vi "Characterizator.vi"(8 "error in (no error)":errorcluster, 11 "Main VI refnums":T4) -> (0 "Error out":errorcluster)   [LabVIEW 2016]
uses:
  Typedefs/Hit chart cluster refnum.ctl
  Typedefs/HitChart refnum.ctl
  <vilib>/Analysis/NI_AALBase.lvlib
panel:
  out "Waveform Chart":T1(graph)
  in  "Tab Control":enum32{"Page 1", "Page 2"}(tab)
  in  "Chnls":enum16{"Chnl 2", "Chnl 1", "Both"}(ring)=enum."Both"
  in  "Begin characterization":bool
  in  "Range max hard":dbl format="%#_g mV"
  in  "Range min hard":dbl format="%#_g mV"
  in  "Levels":i32
  in  "Save path":path=path "D:/Data/Characterizations/Coincidence rate characterizations"
  in  "Scintillator ID":i32
  in  "MPPC Serial number":i32
  in  "ROB 1 ID":i32 caption="ROB ID"
  in  "MPPC Bias":dbl
  in  "Recommended at 25C":bool
  in  "finish level":bool
  out "Current\n trigger level":dbl
  out "Level number":i32
  out "Datapoints ch1":i32
  out "Trigger level \nincrement":dbl
  out "Previous\n trigger level":dbl
  out "Ch1WaveformData":T2
  in  "Scintillator ID":i32
  in  "MPPC Serial number":i32
  in  "ROB 2 ID":i32 caption="ROB ID"
  in  "MPPC Bias":dbl
  in  "Recommended at 25C":bool
  in  "Channel 1":u8 max=15
  in  "Channel 2":u8=1 max=15
  in  "Register for channel events":bool
  out "Ch2WaveformData":T2
  in  "Hard-set trig lvl":bool=TRUE
  in  "Range max perc.":dbl min=0.0 max=100.0 format="%#_g %"
  in  "Range min perc.":dbl min=0.0 max=100.0 format="%#_g %"
  out "Datapoints ch2":i32
  in  "Datapoints to collect":i32=15
  in  "Period (s)":dbl=1.0 format="%#_13g"
  in  "Window(ns)":i32=5
  in  "stop":bool
  out "Command Queue":string[](array[string])
  in  "Data ch1":i32[][](array[numeric])
  out "Range max ref":refnum<vi>
  out "Range min ref":refnum<vi>
  in  "Data ch2":i32[][](array[numeric])
  out "Take data":bool
  in  "generate error":bool
  # "Channel 1"
  # "Channel 2"
  # "(Make sure they match main VI...)"
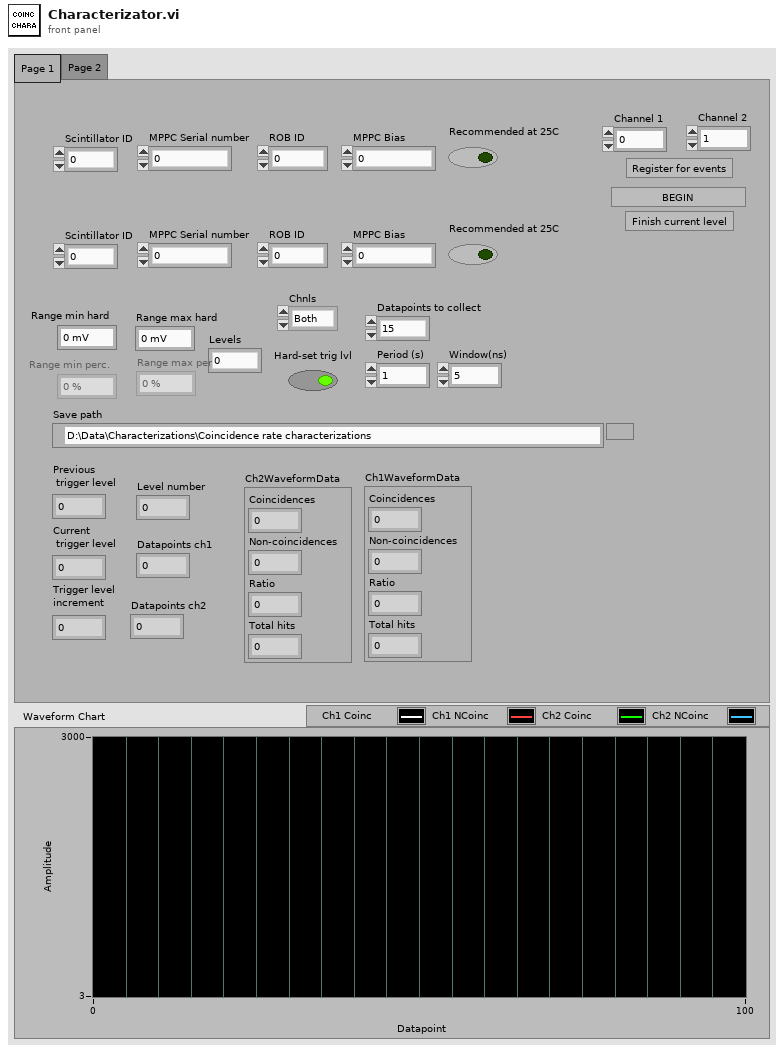
[diagram p1: front panel]
types:
  T1 = cluster{"Ch1 coinc":dbl, "Ch1 Ncoinc":dbl, "Ch2 coinc":dbl, "Ch2 Ncoinc":dbl}
  T2 = cluster{"Coincidences":dbl, "Non-coincidences":dbl, "Ratio":dbl, "Total hits":dbl}
  T3 = typedef "Hit chart cluster refnum.ctl" = refnum<vi>
  T4 = cluster{"VTrig mV":refnum<vi>, "Top hit charts":T3, "Bottom hit charts":T3, "Board selector":refnum<vi>, "VTrig percent ":refnum<vi>, "Hard-set value":refnum<vi>, "Programmatic set trigthres":refnum<vi>}
  T5 = enum16{"open", "replace", "create", "open or create", "replace or create", "replace or create with confirmation"}
  T6 = cluster{"Coincidences":dbl, "Non-coincidences":dbl, "Ratio":dbl, "Total hits":dbl}[]
  T7 = typedef "HitChart refnum.ctl" = refnum<vi>
  T8 = enum8{"Enabled", "Disabled", "Disabled and Grayed Out"}
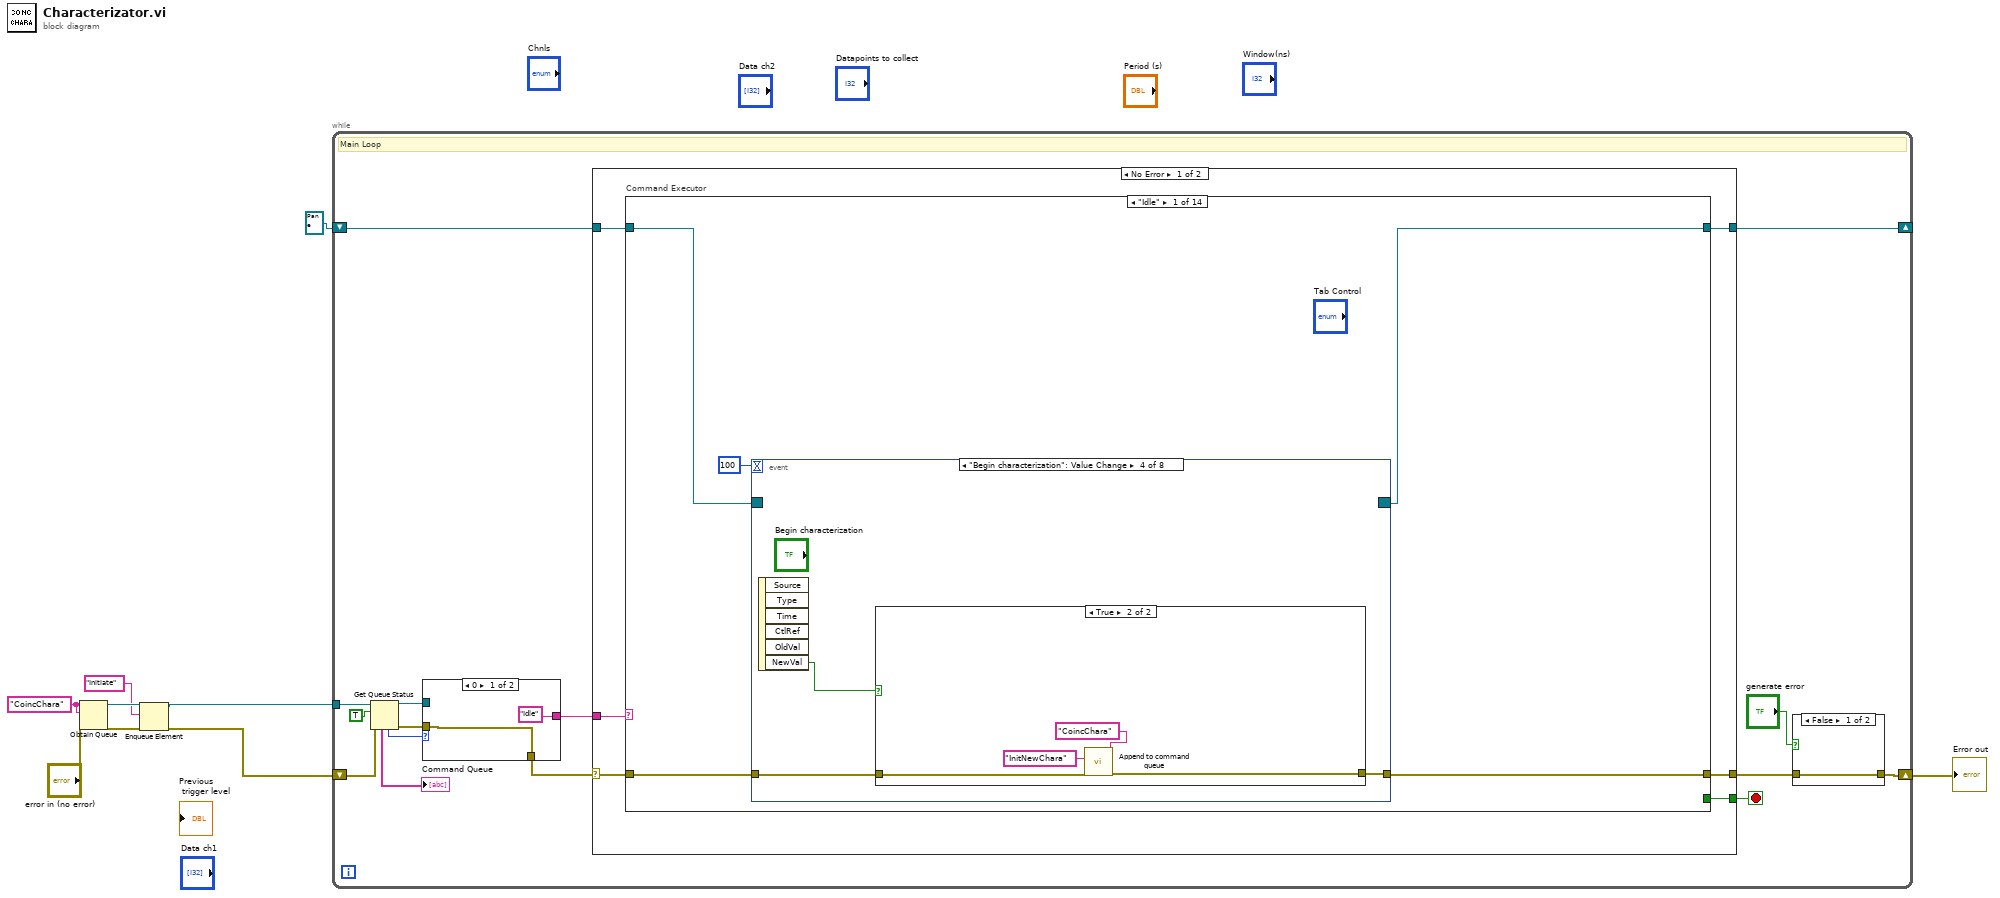
[diagram p0: block diagram]
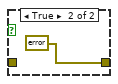
[diagram p2: hidden frame]
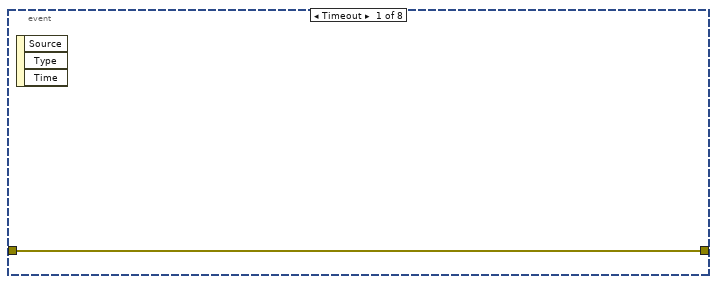
[diagram p3: hidden frame]
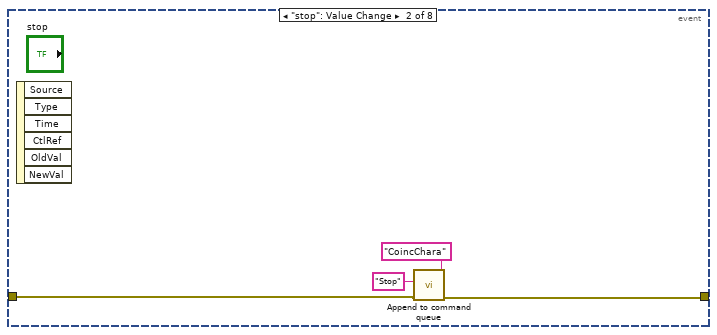
[diagram p4: hidden frame]
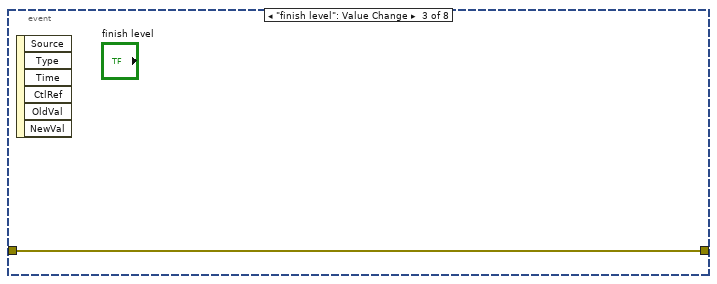
[diagram p5: hidden frame]
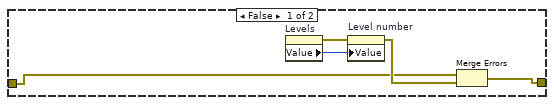
[diagram p6: hidden frame]
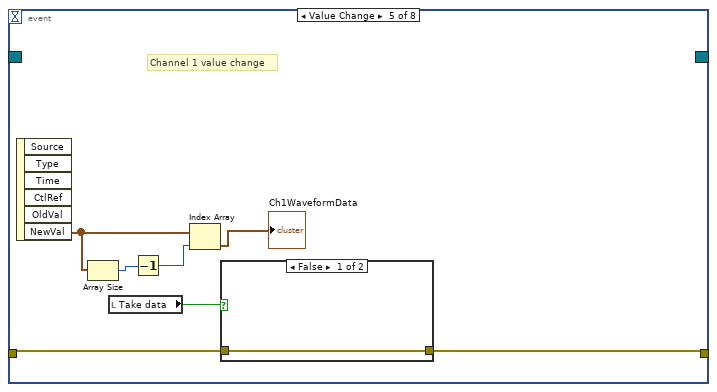
[diagram p7: hidden frame]
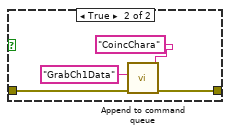
[diagram p8: hidden frame]
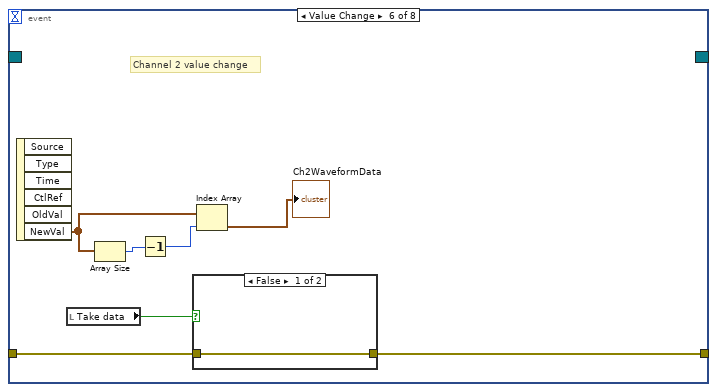
[diagram p9: hidden frame]
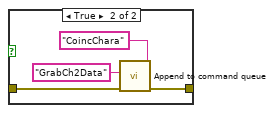
[diagram p10: hidden frame]
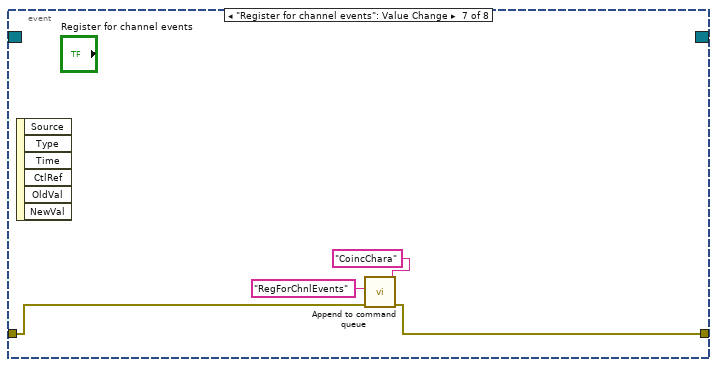
[diagram p11: hidden frame]
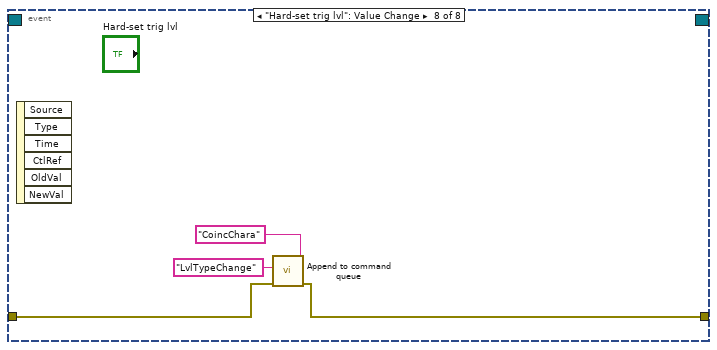
[diagram p12: hidden frame]
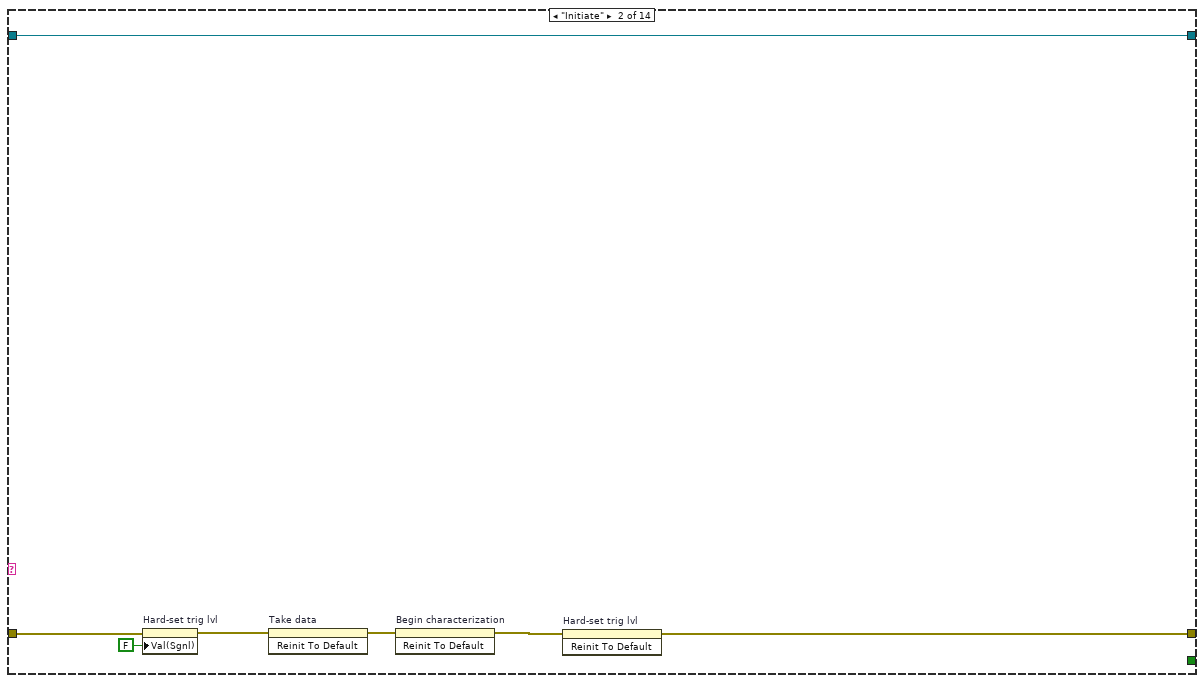
[diagram p13: hidden frame]
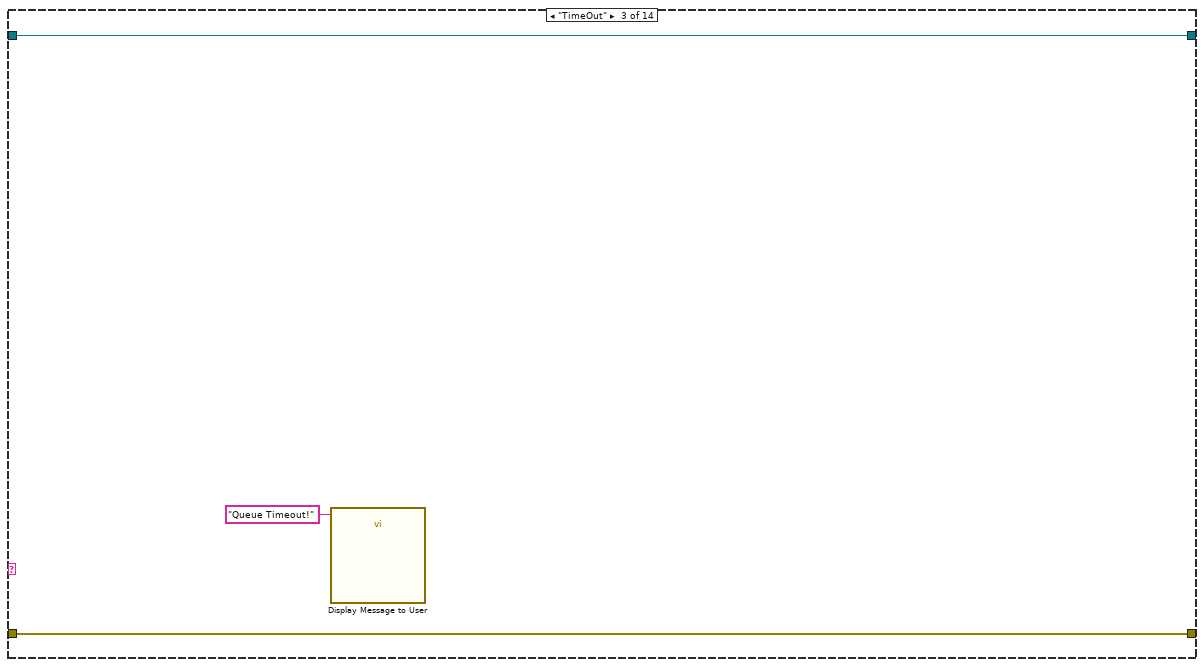
[diagram p14: hidden frame]
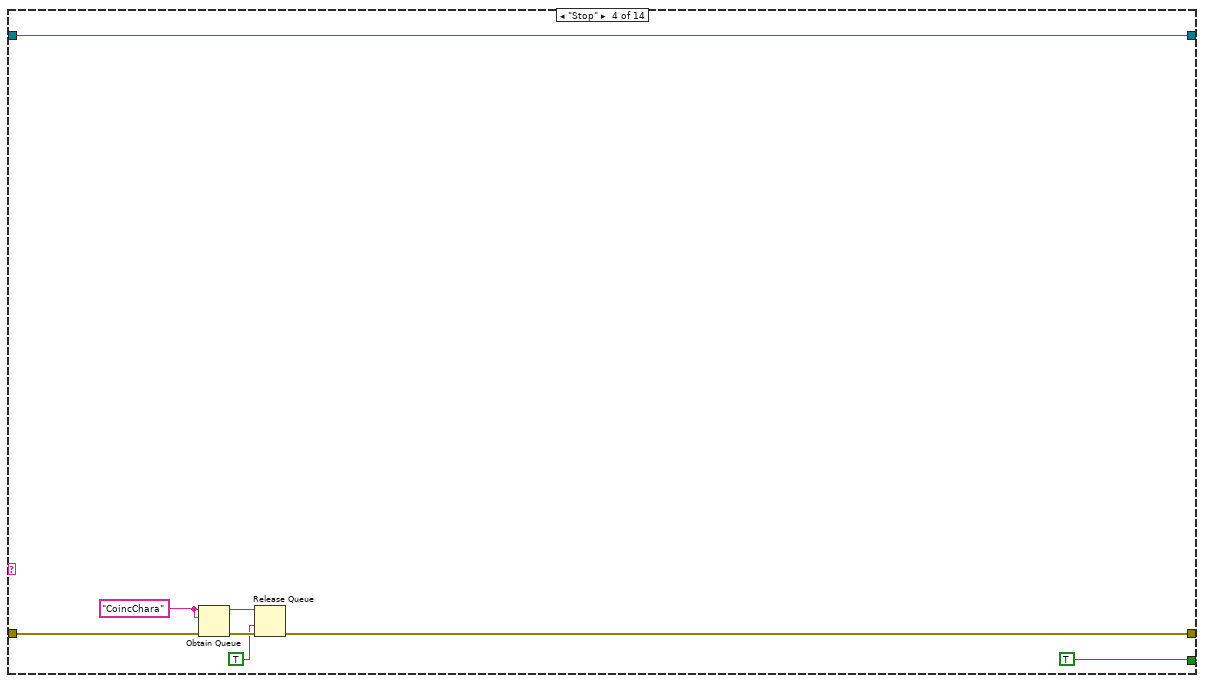
[diagram p15: hidden frame]
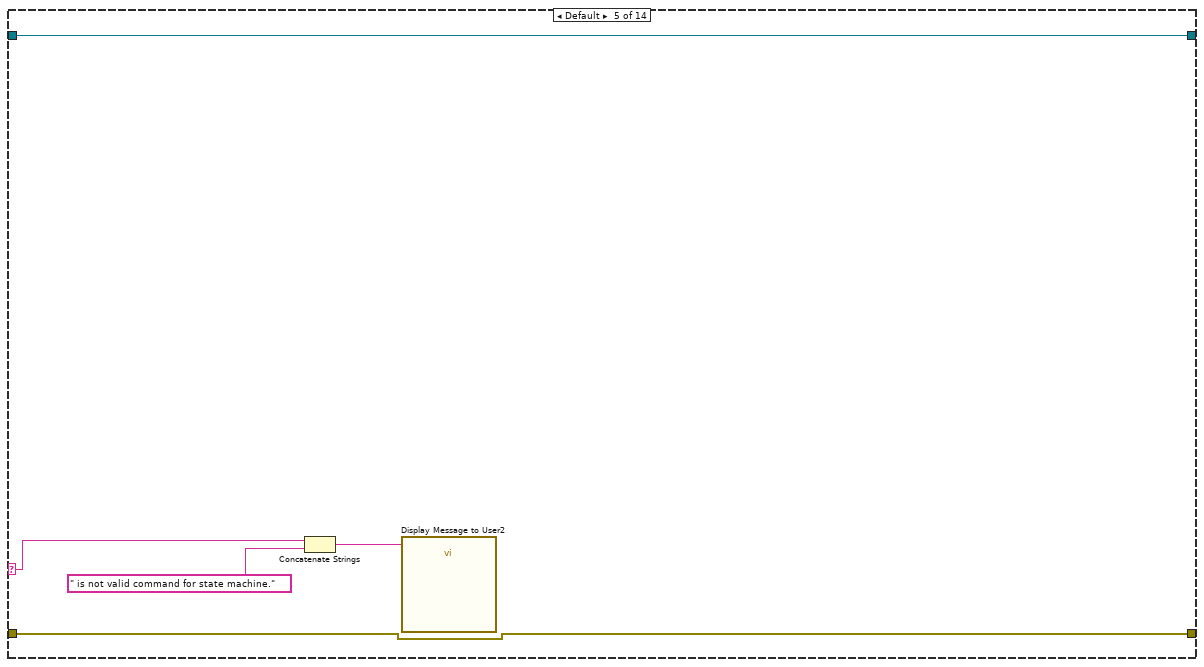
[diagram p16: hidden frame]
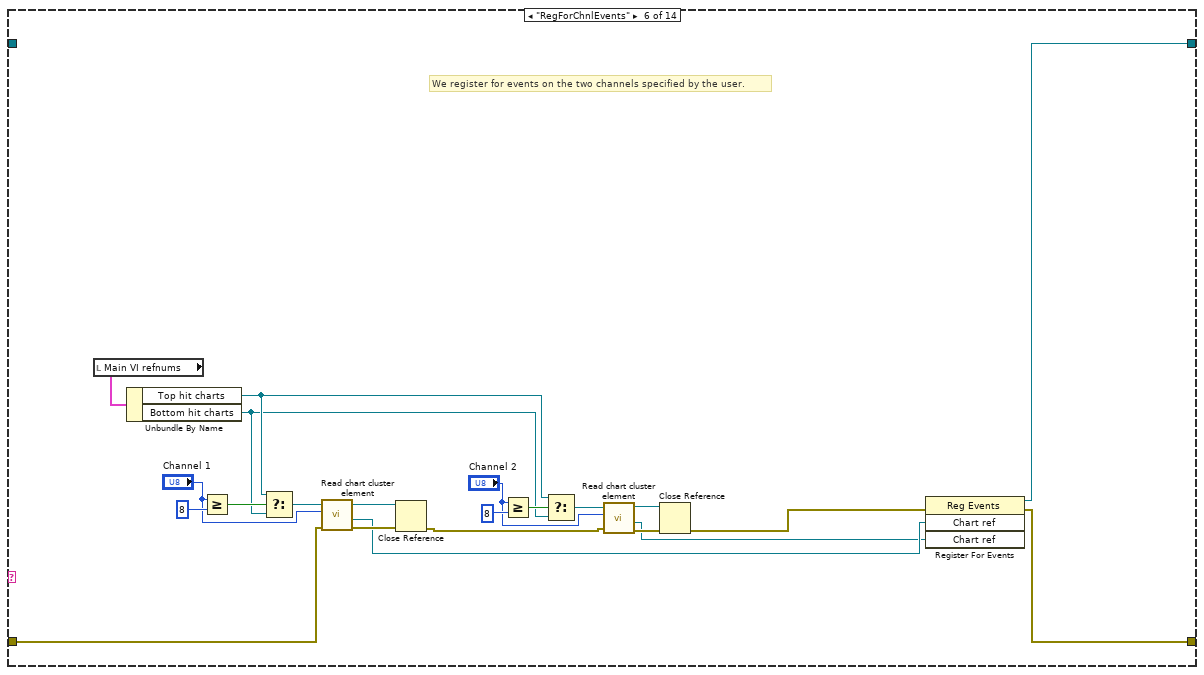
[diagram p17: hidden frame]
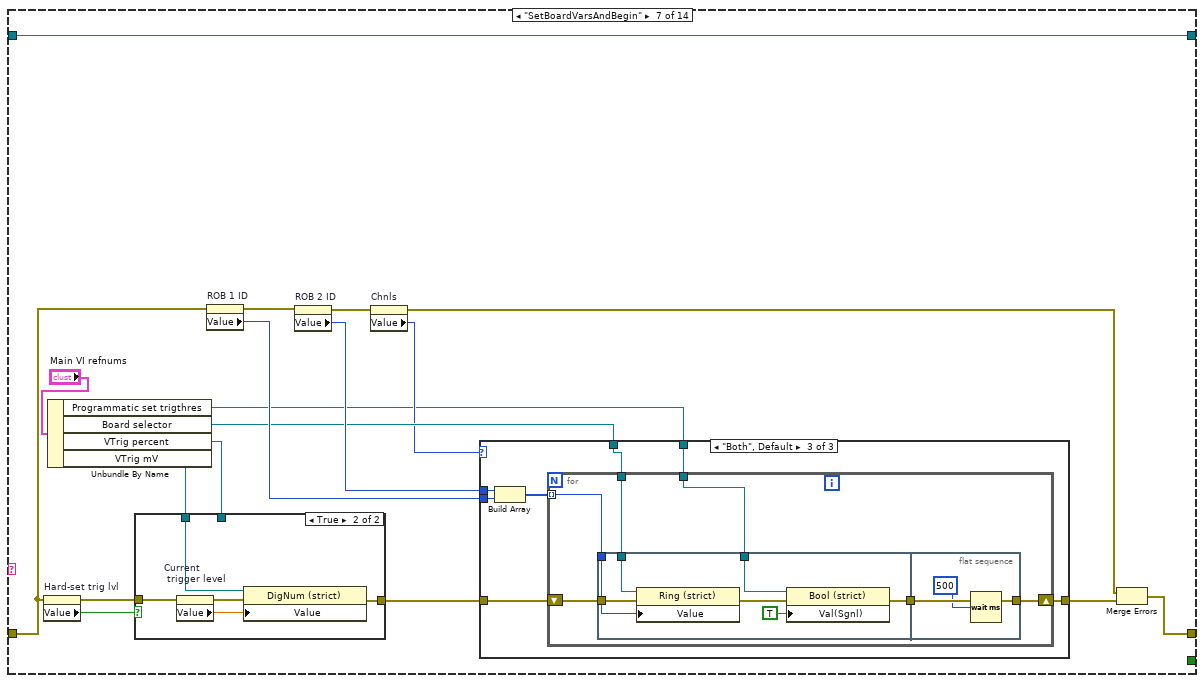
[diagram p18: hidden frame]
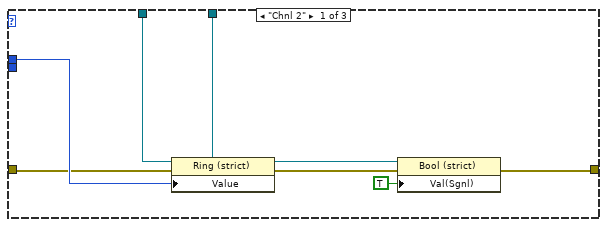
[diagram p19: hidden frame]
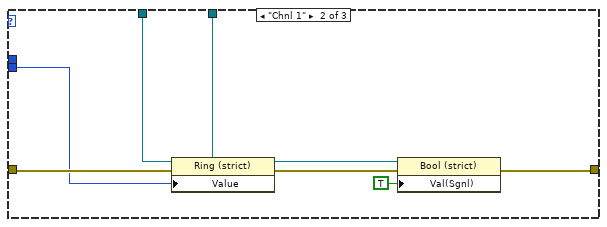
[diagram p20: hidden frame]
diagram:
  w9 = "CoincChara" ("name (unnamed)")
  n1 = Obtain Queue(name (unnamed)=w9, element data type=w9, error in (no error)="error in (no error)") -> (queue out=w7:refnum<queue>, error out=w5:errorcluster)  [unwired: 2 in, 1 out]
  n2 = Enqueue Element(queue=w7, element="Initiate", error in (no error)=w5) -> (queue out=w3:refnum<queue>, error out=w4:errorcluster)  [unwired: 1 in, 1 out]
  n3 = while {
    tunnel: w3 -> [w20]
    shift-right: [w12] -> w2
    shift-left: w4 -> [w17]
    shift-right: [w13] -> _
    shift-left: refnum<event-registration> refnum ("event registration refnum") -> [w14]
    stop <- w16 stop-if-true
    # "Main Loop"
    n4 = Get Queue Status(queue=w20, return elements? (F)=TRUE, error in (no error)=w17) -> (queue out=w23:refnum<queue>, error out=w22:errorcluster, # elements in queue=w24:i32, elements=→"Command Queue":string[])  [unwired: 4 out]
    n5 = case shown="0" w24 {
      tunnel: ["Idle" ("element") w510] -> w18
      tunnel: w23 -> [_ w516]
      tunnel: w22 -> [w506 w515]
      tunnel: [w506 w509] -> w15
      frame 0 {
      }
      frame Default {
        n6 = Dequeue Element(queue=w516, timeout in ms (-1)=50, error in (no error)=w515) -> (element=w514:string, timed out?=w513:bool, error out=w509:errorcluster)  [unwired: 1 out]
        n7 = Not(x=w513) -> (.not. x?=w512:bool)
        n8 = Select(t=w514, s=w512, f="TimeOut") -> (s? t:f=w510:string)
      }
    }
    n9 = case shown="No Error" w15 {
      selector: w15 -> [w29 w499]
      tunnel: w18 -> [w32 _]
      tunnel: [w31 w498] -> w11
      tunnel: [w30 TRUE] -> w16
      tunnel: w14 -> [w28 w495]
      tunnel: [w27 w495] -> w13
      frame No Error {
        n10 = case "Command Executor" shown="\"Idle\"" w32 {
          selector: w32 -> [_ _ _ _ w108 _ _ _ _ _ _ _ _ _]
          tunnel: [w35 w88 w96 w99 w107 w115 w141 w211 w225 w317 w374 w391 w406 w450] -> w31
          tunnel: w29 -> [w36 w92 w96 w100 w107 w116 w143 w200 w227 w271 w381 w394 w422 w467]
          tunnel: [_ _ _ TRUE _ _ _ _ _ _ _ _ _ _] -> w30
          tunnel: w28 -> [w34 w94 w95 w98 w106 _ w150 w208 w217 w314 w379 w404 w418 w463]
          tunnel: [w33 w94 w95 w98 w106 w114 w150 w208 w217 w314 w379 w404 w418 w463] -> w27
          frame "Idle" {
            n11 = event shown="[3] \"Begin characterization\": Value Change" {
              selector: w34 -> [_ _ _ _ _ _ _ _]
              dyn-events: [_ _ _ _ _ _ _ _] -> w33
              timeout: 100 -> [_ _ _ _ _ _ _ _]
              tunnel: w36 -> [w38 w42 w43 w46 w62 w74 w81 w86]
              tunnel: [w38 w41 w43 w45 w61 w73 w80 w85] -> w35
              event Timeout {
                n12 = event-data() -> ()  [unwired: 1 in, 3 out]
              }
              event "stop": Value Change {
                n13 = event-data() -> ()  [unwired: 1 in, 6 out]
                n14 = call "Append to command queue.vi"("Name (CommandQueue)"="CoincChara", "error in (no error)"=w42, "Single command"="Stop") -> ("error out"=w41:errorcluster)  [unwired: 8 in]
              }
              event "finish level": Value Change {
                n15 = event-data() -> ()  [unwired: 1 in, 6 out]
              }
              event "Begin characterization": Value Change {
                n16 = event-data() -> ("NewVal"=w44:bool)  [unwired: 1 in, 5 out]
                n17 = case shown="True" w44 {
                  tunnel: w46 -> [w47 w54]
                  tunnel: [w48 w53] -> w45
                  frame False {
                    n18 = property on="Levels" class="DigNum (strict)"() -> (error out=w50:errorcluster, "Value"=w51:i32)  [unwired: 2 in, 1 out]
                    n19 = property on="Level number" class="DigNum (strict)"(error in=w50, "Value"=w51) -> (error out=w49:errorcluster)  [unwired: 1 in, 1 out]
                    n20 = Merge Errors(w47, w49) -> (w48:errorcluster)
                  }
                  frame True {
                    n21 = call "Append to command queue.vi"("Name (CommandQueue)"="CoincChara", "error in (no error)"=w54, "Single command"="InitNewChara") -> ("error out"=w53:errorcluster)  [unwired: 8 in]
                  }
                }
              }
              event Value Change {
                # "Channel 1 value change"
                n22 = event-data() -> ("NewVal"=w58:T6)  [unwired: 1 in, 5 out]
                n23 = Array Size(array=w58) -> (size(s)=w57:i32)
                n24 = local read "Take data"() -> (w60:bool)
                n25 = Decrement(x=w57) -> (x-1=w56:i32)
                n26 = Index Array(array=w58, index=w56) -> (element=→"Ch1WaveformData":T2)
                n27 = case shown="False" w60 {
                  tunnel: w62 -> [w63 w65]
                  tunnel: [w63 w64] -> w61
                  frame False {
                  }
                  frame True {
                    n28 = call "Append to command queue.vi"("Name (CommandQueue)"="CoincChara", "error in (no error)"=w65, "Single command"="GrabCh1Data") -> ("error out"=w64:errorcluster)  [unwired: 8 in]
                  }
                }
              }
              event Value Change {
                # "Channel 2 value change"
                n29 = event-data() -> ("NewVal"=w69:T6)  [unwired: 1 in, 5 out]
                n30 = local read "Take data"() -> (w72:bool)
                n31 = Array Size(array=w69) -> (size(s)=w71:i32)
                n32 = Decrement(x=w71) -> (x-1=w70:i32)
                n33 = case shown="False" w72 {
                  tunnel: w74 -> [w75 w78]
                  tunnel: [w75 w77] -> w73
                  frame False {
                  }
                  frame True {
                    n34 = call "Append to command queue.vi"("Name (CommandQueue)"="CoincChara", "error in (no error)"=w78, "Single command"="GrabCh2Data") -> ("error out"=w77:errorcluster)  [unwired: 8 in]
                  }
                }
                n35 = Index Array(array=w69, index=w70) -> (element=→"Ch2WaveformData":T2)
              }
              event "Register for channel events": Value Change {
                n36 = event-data() -> ()  [unwired: 1 in, 6 out]
                n37 = call "Append to command queue.vi"("Name (CommandQueue)"="CoincChara", "error in (no error)"=w81, "Single command"="RegForChnlEvents") -> ("error out"=w80:errorcluster)  [unwired: 8 in]
              }
              event "Hard-set trig lvl": Value Change {
                n38 = event-data() -> ()  [unwired: 1 in, 6 out]
                n39 = call "Append to command queue.vi"("Name (CommandQueue)"="CoincChara", "error in (no error)"=w86, "Single command"="LvlTypeChange") -> ("error out"=w85:errorcluster)  [unwired: 8 in]
              }
            }
          }
          frame "Initiate" {
            n40 = property on="Hard-set trig lvl" class="Bool (strict)"(error in=w92, "Val(Sgnl)"=FALSE ("Value (Signaling)")) -> (error out=w91:errorcluster)  [unwired: 1 in, 1 out]
            n41 = invoke on="Take data" class="Bool (strict)" method="Reinit To Default"(error in=w91) -> (error out=w90:errorcluster)  [unwired: 2 in, 2 out]
            n42 = invoke on="Begin characterization" class="Bool (strict)" method="Reinit To Default"(error in=w90) -> (error out=w89:errorcluster)  [unwired: 2 in, 2 out]
            n43 = invoke on="Hard-set trig lvl" class="Bool (strict)" method="Reinit To Default"(error in=w89) -> (error out=w88:errorcluster)  [unwired: 2 in, 2 out]
          }
          frame "TimeOut" {
            n44 = call "Display Message to User"("Message"="Queue Timeout!" ("string")) -> ()  [unwired: 9 in, 2 out]
          }
          frame "Stop" {
            w101 = "CoincChara" ("name (unnamed)")
            n45 = Obtain Queue(name (unnamed)=w101, element data type=w101, error in (no error)=w100) -> (queue out=w104:refnum<queue>, error out=w103:errorcluster)  [unwired: 2 in, 1 out]
            n46 = Release Queue(queue=w104, force destroy? (F)=TRUE, error in (no error)=w103) -> (error out=w99:errorcluster)  [unwired: 2 out]
          }
          frame Default {
            n47 = Concatenate Strings(w108, " is not valid command for state machine." ("string")) -> (w109:string)
            n48 = call "Display Message to User2"("Message"=w109) -> ()  [unwired: 9 in, 2 out]
          }
          frame "RegForChnlEvents" {
            # "We register for events on the two channels specified by the user."
            n49 = local read "Main VI refnums"() -> (w113:T4)
            n50 = Unbundle By Name(w113) -> ("Top hit charts"=w112:T3, "Bottom hit charts"=w111:T3)
            n51 = Greater Or Equal?(x="Channel 1", y=u8 8) -> (x >= y?=w131:bool)
            n52 = Select(t=w112, s=w131, f=w111) -> (s? t:f=w130:T3)
            n53 = call "Read chart cluster element.vi"("error in (no error)"=w116, "Channel"="Channel 1", "Chart cluster"=w130) -> ("error out"=w124:errorcluster, "Chart ref"=w118:T7, "Chart cluster"=w123:T3)  [unwired: 5 in, 1 out]
            n54 = Close Reference(reference=w123, error in (no error)=w124) -> (error out=w122:errorcluster)
            n55 = Greater Or Equal?(x="Channel 2", y=u8 8) -> (x >= y?=w127:bool)
            n56 = Select(t=w112, s=w127, f=w111) -> (s? t:f=w128:T3)
            n57 = call "Read chart cluster element.vi"("error in (no error)"=w122, "Channel"="Channel 2", "Chart cluster"=w128) -> ("error out"=w121:errorcluster, "Chart ref"=w117:T7, "Chart cluster"=w119:T3)  [unwired: 5 in, 1 out]
            n58 = Close Reference(reference=w119, error in (no error)=w121) -> (error out=w120:errorcluster)
            n59 = register-events(error in=w120, w118, w117) -> (reference out=w114:refnum<event-registration>, error out=w115:errorcluster)  [unwired: 1 in]
          }
          frame "SetBoardVarsAndBegin" {
            n60 = property on="Hard-set trig lvl" class="Bool (strict)"(error in=w143) -> (error out=w147:errorcluster, "Value"=w148:bool)  [unwired: 1 in, 1 out]
            n61 = Unbundle By Name("Main VI refnums") -> ("Programmatic set trigthres"=w133:refnum<vi>, "Board selector"=w140:refnum<vi>, "VTrig percent"=w139:refnum<vi>, "VTrig mV"=w138:refnum<vi>)
            n62 = case shown="True" w148 {
              tunnel: [w189 w194] -> w149
              tunnel: w147 -> [w188 w193]
              tunnel: w139 -> [w187 _]
              tunnel: w138 -> [_ w192]
              frame False {
                n63 = property on="Current\n trigger level" class="DigNum (strict)"(error in=w188) -> (error out=w190:errorcluster, "Value"=w191:dbl)  [unwired: 1 in, 1 out]
                n64 = property class="DigNum (strict)"(reference=w187, error in=w190, "Value"=w191) -> (error out=w189:errorcluster)  [unwired: 1 out]
              }
              frame True {
                n65 = property on="Current\n trigger level" class="DigNum (strict)"(error in=w193) -> (error out=w195:errorcluster, "Value"=w196:dbl)  [unwired: 1 in, 1 out]
                n66 = property class="DigNum (strict)"(reference=w192, error in=w195, "Value"=w196) -> (error out=w194:errorcluster)  [unwired: 1 out]
              }
            }
            n67 = property on="ROB 1 ID" class="DigNum (strict)"(error in=w143) -> (error out=w146:errorcluster, "Value"=w144:i32)  [unwired: 1 in, 1 out]
            n68 = property on="ROB 2 ID" class="DigNum (strict)"(error in=w146) -> (error out=w137:errorcluster, "Value"=w145:i32)  [unwired: 1 in, 1 out]
            n69 = property on="Chnls" class="Enum (strict)"(error in=w137) -> (error out=w136:errorcluster, "Value"=w135:enum16{"Chnl 2", "Chnl 1", "Both"})  [unwired: 1 in, 1 out]
            n70 = case shown="\"Both\", Default" w135 {
              tunnel: w149 -> [w151 w159 w171]
              tunnel: w145 -> [w152 _ w170]
              tunnel: w144 -> [_ w158 w169]
              tunnel: [w155 w162 w167] -> w142
              tunnel: w140 -> [w153 w160 w166]
              tunnel: w133 -> [w154 w161 w165]
              frame "Chnl 2" {
                n71 = property class="Ring (strict)"(reference=w153, error in=w151, "Value"=w152) -> (error out=w156:errorcluster)  [unwired: 1 out]
                n72 = property class="Bool (strict)"(reference=w154, error in=w156, "Val(Sgnl)"=TRUE ("Value (Signaling)")) -> (error out=w155:errorcluster)  [unwired: 1 out]
              }
              frame "Chnl 1" {
                n73 = property class="Ring (strict)"(reference=w160, error in=w159, "Value"=w158) -> (error out=w163:errorcluster)  [unwired: 1 out]
                n74 = property class="Bool (strict)"(reference=w161, error in=w163, "Val(Sgnl)"=TRUE ("Value (Signaling)")) -> (error out=w162:errorcluster)  [unwired: 1 out]
              }
              frame "Both", Default {
                n75 = Build Array(w170, w169) -> (w168:i32[])
                n76 = for {
                  tunnel: w166 -> [w175]
                  tunnel: w165 -> [w174]
                  tunnel: w168 -> [w173] mode=indexing
                  shift-right: [w177] -> w167
                  shift-left: w171 -> [w176]
                  n77 = flat-sequence {
                    tunnel: w176 -> [w182]
                    tunnel: w175 -> [w180]
                    tunnel: w174 -> [w179]
                    tunnel: w173 -> [w178]
                    tunnel: [w183] -> w172
                    tunnel: [w186] -> w177
                    tunnel: w172 -> [w186]
                    frame #0 {
                      n78 = property class="Ring (strict)"(reference=w180, error in=w182, "Value"=w178) -> (error out=w181:errorcluster)  [unwired: 1 out]
                      n79 = property class="Bool (strict)"(reference=w179, error in=w181, "Val(Sgnl)"=TRUE ("Value (Signaling)")) -> (error out=w183:errorcluster)  [unwired: 1 out]
                    }
                    frame #1 {
                      n80 = Wait (ms)(milliseconds to wait=500) -> ()  [unwired: 1 out]
                    }
                  }
                }
              }
            }
            n81 = Merge Errors(w136, w142) -> (w141:errorcluster)
          }
          frame "InitNewChara" {
            w198 = -2 ("Datapoints")
            n82 = property on="Range min ref" class="LVObjRef (strict)"(error in=w200) -> (error out=w203:errorcluster, "Value"=w204:refnum<vi>)  [unwired: 1 in, 1 out]
            n83 = property class="DigNum (strict)"(reference=w204, error in=w203) -> (error out=w201:errorcluster, "Value"=w206:dbl)  [unwired: 1 out]
            n84 = property on="Range max ref" class="LVObjRef (strict)"(error in=w201) -> (error out=w202:errorcluster, "Value"=w205:refnum<vi>)  [unwired: 1 in, 1 out]
            n85 = property class="DigNum (strict)"(reference=w205, error in=w202) -> (error out=w199:errorcluster, "Value"=w207:dbl)  [unwired: 1 out]
            "Current\n trigger level" <- w207
            n86 = Decrement(x="Levels") -> (x-1=w209:i32)
            n87 = local write "Take data"(TRUE ("Take data")) -> ()
            n88 = Subtract(x=w207, y=w206) -> (x-y=w215:dbl)
            n89 = Divide(x=w215, y=w209) -> (x/y=→"Trigger level \nincrement":dbl)
            n90 = call "Append to command queue.vi"("Name (CommandQueue)"="CoincChara", "error in (no error)"=w199, "Single command"="SetBoardVarsAndBegin") -> ("error out"=w211:errorcluster)  [unwired: 8 in]
            "Level number" <- 1 ("Level number")
            "Datapoints ch1" <- w198
            "Datapoints ch2" <- w198
          }
          frame "LevelDone" {
            n91 = property on="Levels" class="DigNum (strict)"(error in=w227) -> (error out=w228:errorcluster, "Value"=w229:i32)  [unwired: 1 in, 1 out]
            n92 = property on="Level number" class="DigNum (strict)"(error in=w228) -> (error out=w222:errorcluster, "Value"=w230:i32)  [unwired: 1 in, 1 out]
            n93 = Equal?(x=w230, y=w229) -> (x = y?=w226:bool)
            n94 = call "Append to command queue.vi"("Name (CommandQueue)"="CoincChara", "error in (no error)"=w222, "Single command"="SaveData") -> ("error out"=w219:errorcluster)  [unwired: 8 in]
            n95 = property on="Current\n trigger level" class="DigNum (strict)"(error in=w219) -> (error out=w220:errorcluster, "Value"=w221:dbl)  [unwired: 1 in, 1 out]
            n96 = property on="Previous\n trigger level" class="DigNum (strict)"(error in=w220, "Value"=w221) -> (error out=w218:errorcluster)  [unwired: 1 in, 1 out]
            n97 = case shown="False" w226 {
              tunnel: w218 -> [w241 w251]
              tunnel: [w231 w250] -> w225
              frame False {
                w236 = -2 ("Datapoints ch1")
                n98 = property on="Trigger level \nincrement" class="DigNum (strict)"(error in=w241) -> (error out=w245:errorcluster, "Value"=w244:dbl)  [unwired: 1 in, 1 out]
                n99 = property on="Current\n trigger level" class="DigNum (strict)"(error in=w245) -> (error out=w242:errorcluster, "Value"=w237:dbl)  [unwired: 1 in, 1 out]
                n100 = Subtract(x=w237, y=w244) -> (x-y=w243:dbl)
                n101 = property on="Current\n trigger level" class="DigNum (strict)"(error in=w242, "Value"=w243) -> (error out=w234:errorcluster)  [unwired: 1 in, 1 out]
                n102 = property on="Level number" class="DigNum (strict)"(error in=w234) -> (error out=w246:errorcluster, "Value"=w248:i32)  [unwired: 1 in, 1 out]
                n103 = property on="Datapoints ch1" class="DigNum (strict)"(error in=w234, "Value"=w236) -> (error out=w235:errorcluster)  [unwired: 1 in, 1 out]
                n104 = property on="Datapoints ch2" class="DigNum (strict)"(error in=w235, "Value"=w236) -> (error out=w233:errorcluster)  [unwired: 1 in, 1 out]
                n105 = Increment(x=w248) -> (x+1=w247:i32)
                n106 = property on="Level number" class="DigNum (strict)"(error in=w246, "Value"=w247) -> (error out=w238:errorcluster)  [unwired: 1 in, 1 out]
                n107 = call "Append to command queue.vi"("Name (CommandQueue)"="CoincChara", "error in (no error)"=w238, "Single command"="SetBoardVarsAndBegin") -> ("error out"=w232:errorcluster)  [unwired: 8 in]
                n108 = Merge Errors(w232, w233) -> (w231:errorcluster)
              }
              frame True {
                n109 = call "Append to command queue.vi"("Name (CommandQueue)"="CoincChara", "error in (no error)"=w251, "Single command"="Reset") -> ("error out"=w250:errorcluster)  [unwired: 8 in]
              }
            }
          }
          frame "SaveData" {
            w275 = i32[][] [] ("Data")
            n110 = property on="Period (s)" class="DigNum (strict)"(error in=w271) -> (error out=w294:errorcluster, "Value"=w295:dbl)  [unwired: 1 in, 1 out]
            n111 = property on="Previous\n trigger level" class="DigNum (strict)"(error in=w294) -> (error out=w277:errorcluster, "Value"=w296:dbl)  [unwired: 1 in, 1 out]
            n112 = property on="Hard-set trig lvl" class="Bool (strict)"(error in=w277) -> (error out=w254:errorcluster, "Value"=w285:bool)  [unwired: 1 in, 1 out]
            n113 = Number To Decimal String(number=w296) -> (decimal integer string=w311:string)  [unwired: 1 in]
            n114 = Number To Decimal String(number=w295) -> (decimal integer string=w315:string)  [unwired: 1 in]
            n115 = call "Build header single level.vi"("Overvoltage"="MPPC Bias", "Recommended at 25C"="Recommended at 25C", "MPPC Serial number"="MPPC Serial number", "ROB ID"="ROB 1 ID", "Scintillator ID"="Scintillator ID") -> ("Header"=w280:string)  [unwired: 6 in]
            n116 = Select(t="percent " ("string"), s=w285, f="mV " ("string")) -> (s? t:f=w286:string)
            n117 = Concatenate Strings(w311, w286, w315, "s.csv " ("string")) -> (w331:string)
            n118 = call "Build header single level.vi"("Overvoltage"="MPPC Bias", "Recommended at 25C"="Recommended at 25C", "Add timestamp"=FALSE, "MPPC Serial number"="MPPC Serial number", "ROB ID"="ROB 2 ID", "Scintillator ID"="Scintillator ID") -> ("Header"=w279:string)  [unwired: 5 in]
            n119 = Build Array(w280, w279) -> (w278:string[])
            n120 = Build Array("Ch1" ("string"), "Ch2" ("string")) -> (w281:string[])
            n121 = Select(t="Hardset" ("string"), s=w285, f="Percent" ("string")) -> (s? t:f=w291:string)
            n122 = Concatenate Strings("Trig lvl:  " ("string"), w291) -> (w289:string)
            n123 = property on="Data ch2" class="Arr (strict)"() -> (error out=w310:errorcluster, "Value"=w269:i32[][])  [unwired: 2 in, 1 out]
            n124 = property on="Data ch1" class="Arr (strict)"(error in=w310) -> (error out=w309:errorcluster, "Value"=w270:i32[][])  [unwired: 1 in, 1 out]
            n125 = Index Array(array=w270, index (col) #1=0 ("index (row)"), index (col) #2=1 ("index (row)")) -> (element #1=w268:i32[], element #2=w267:i32[])  [unwired: 2 in]
            n126 = Index Array(array=w269, index (col) #1=0 ("index (row)"), index (col) #2=1 ("index (row)")) -> (element #1=w266:i32[], element #2=w265:i32[])  [unwired: 2 in]
            n127 = Build Array(w270, w269) -> (w276:i32[][][])
            n128 = for {
              N: 2 -> [_]
              tunnel: "Save path" -> [w342]
              tunnel: w331 -> [w351]
              tunnel: w281 -> [w341] mode=indexing
              tunnel: w278 -> [w340] mode=indexing
              tunnel: w276 -> [w339] mode=indexing
              shift-right: [w343] -> w253
              shift-left: w254 -> [w337]
              n129 = Build Path(base path=w342, name or relative path=w341) -> (appended path=w338:path)
              n130 = call "Find or make folder.vi"("error in"=w337, "Folder to find/make"=w338) -> ("error out"=w336:errorcluster, "created path"=w335:path)  [unwired: 7 in, 1 out]
              n131 = Build Path(base path=w335, name or relative path=w351) -> (appended path=w353:path)
              n132 = Open/Create/Replace File(file path (use dialog)=w353, error in=w336, operation (0:open)=T5."open or create") -> (refnum out=w348:refnum<file>, error out=w347:errorcluster)  [unwired: 3 in, 1 out]
              n133 = Array To Spreadsheet String(delimiter (Tab)="\t", array=w339, 3:"%d" ("format string")) -> (spreadsheet string=w349:string)
              n134 = Concatenate Strings(w340, w349) -> (w346:string)
              n135 = Write to Text File(file (use dialog)=w348, text=w346, error in=w347) -> (refnum out=w345:refnum<file>, error out=w344:errorcluster)  [unwired: 1 in, 1 out]
              n136 = Close File(refnum=w345, error in=w344) -> (error out=w343:errorcluster)  [unwired: 1 out]
            }
            n137 = property on="Save path" class="Path"(error in=w253) -> (error out=w318:errorcluster, "Value"=w329:path)  [unwired: 1 in, 1 out]
            n138 = Build Path(base path=w329, name or relative path="Summary.csv") -> (appended path=w324:path)
            n139 = Open/Create/Replace File(file path (use dialog)=w324, error in=w318, operation (0:open)=T5."open") -> (refnum out=w327:refnum<file>, error out=w326:errorcluster)  [unwired: 3 in, 1 out]
            n140 = Unbundle By Name(w326) -> ("code"=w325:i32)
            n141 = case shown="7" w325 {
              tunnel: w327 -> [_ w372]
              tunnel: w326 -> [_ w371]
              tunnel: w324 -> [w364 _]
              tunnel: [w361 w367] -> w322
              tunnel: [w360 w366] -> w323
              tunnel: w279 -> [w357 _]
              tunnel: w280 -> [w356 _]
              tunnel: w289 -> [w355 _]
              frame 7 {
                w354 = "\r\n"
                n142 = call "Summary header gen.vi"() -> ("Header"=w358:string)
                n143 = Open/Create/Replace File(file path (use dialog)=w364, operation (0:open)=T5."create") -> (refnum out=w362:refnum<file>, error out=w363:errorcluster)  [unwired: 4 in, 1 out]
                n144 = Concatenate Strings(w356, w357, w358, w354, w355, w354) -> (w359:string)
                n145 = Write to Text File(file (use dialog)=w362, text=w359, error in=w363) -> (refnum out=w361:refnum<file>, error out=w360:errorcluster)  [unwired: 1 in, 1 out]
              }
              frame Default {
                n146 = Get File Size(file=w372, error in=w371) -> (refnum out=w370:refnum<file>, size (in bytes)=w369:i64, 0:w368:errorcluster)
                n147 = Set File Position(offset (in bytes) (0)=w369, refnum=w370, error in=w368) -> (refnum out=w367:refnum<file>, error out=w366:errorcluster)  [unwired: 1 in]
              }
            }
            n148 = call <vilib>:"Std Deviation and Variance.vi"("X"=w268) -> ("mean"=w263:dbl)  [unwired: 1 in, 2 out]
            n149 = call <vilib>:"Std Deviation and Variance.vi"("X"=w267) -> ("mean"=w262:dbl)  [unwired: 1 in, 2 out]
            n150 = call <vilib>:"Std Deviation and Variance.vi"("X"=w266) -> ("mean"=w261:dbl)  [unwired: 1 in, 2 out]
            n151 = call <vilib>:"Std Deviation and Variance.vi"("X"=w265) -> ("mean"=w260:dbl)  [unwired: 1 in, 2 out]
            n152 = property on="Period (s)" class="DigNum (strict)"(error in=w309) -> (error out=w308:errorcluster, "Value"=w313:dbl)  [unwired: 1 in, 1 out]
            n153 = Bundle By Name(cluster=T1 {"Ch1 coinc"=0.0, "Ch1 Ncoinc"=0.0, "Ch2 coinc"=0.0, "Ch2 Ncoinc"=0.0} ("Waveform Chart"), "Ch1 coinc"=w263, "Ch1 Ncoinc"=w262, "Ch2 coinc"=w261, "Ch2 Ncoinc"=w260) -> (→"Waveform Chart":T1)
            n154 = property on="Window(ns)" class="DigNum (strict)"(error in=w308) -> (error out=w272:errorcluster, "Value"=w312:i32)  [unwired: 1 in, 1 out]
            n155 = call "Data to sumamry.vi"("Window (ns)"=w312, "Period (seconds)"=w313, "Trig lvl"=w311, "ch2 data"=w269, "ch1 data"=w270) -> ("String out"=w321:string)  [unwired: 6 in]
            n156 = Write to Text File(file (use dialog)=w322, text=w321, error in=w323) -> (refnum out=w319:refnum<file>, error out=w320:errorcluster)  [unwired: 1 in, 1 out]
            n157 = property on="Data ch1" class="Arr (strict)"(error in=w272, "Value"=w275) -> (error out=w274:errorcluster)  [unwired: 1 in, 1 out]
            n158 = property on="Data ch2" class="Arr (strict)"(error in=w274, "Value"=w275) -> (error out=w273:errorcluster)  [unwired: 1 in, 1 out]
            n159 = Close File(refnum=w319, error in=w320) -> (error out=w316:errorcluster)  [unwired: 1 out]
            n160 = Merge Errors(w316, w273) -> (w317:errorcluster)
          }
          frame "Reset" {
            w377 = -2 ("Datapoints")
            n161 = property on="Level number" class="DigNum (strict)"(error in=w381, "Value"=1 ("Level number")) -> (error out=w380:errorcluster)  [unwired: 1 in, 1 out]
            n162 = property on="Datapoints ch1" class="DigNum (strict)"(error in=w380, "Value"=w377) -> (error out=w378:errorcluster)  [unwired: 1 in, 1 out]
            n163 = property on="Datapoints ch2" class="DigNum (strict)"(error in=w378, "Value"=w377) -> (error out=w375:errorcluster)  [unwired: 1 in, 1 out]
            n164 = property on="Begin characterization" class="Bool (strict)"(error in=w375, "Value"=FALSE ("Begin characterization")) -> (error out=w374:errorcluster)  [unwired: 1 in, 1 out]
            "Take data" <- FALSE ("Boolean")
          }
          frame "LvlTypeChange" {
            w399 = T8."Disabled and Grayed Out" ("Disabled")
            w400 = T8."Enabled" ("Disabled")
            n165 = property on="Hard-set trig lvl" class="Bool (strict)"(error in=w394) -> (error out=w398:errorcluster, "Value"=w395:bool)  [unwired: 1 in, 1 out]
            n166 = local read "Main VI refnums"() -> (w388:T4)
            n167 = Unbundle By Name(w388) -> ("Hard-set value"=w387:refnum<vi>)
            n168 = Select(t=w400, s=w395, f=w399) -> (s? t:f=w397:T8)
            n169 = property class="Bool (strict)"(reference=w387, error in=w394, "Val(Sgnl)"=w395) -> (error out=w392:errorcluster)  [unwired: 1 out]
            n170 = Select(t=w399, s=w395, f=w400) -> (s? t:f=w396:T8)
            n171 = control-ref of="Range max hard"() -> (w386:refnum<vi>)
            n172 = property class="DigNum (strict)"(reference=w386, error in=w398, "DisabledEnum"=w397) -> (error out=w403:errorcluster)  [unwired: 1 out]
            n173 = control-ref of="Range min hard"() -> (w383:refnum<vi>)
            n174 = property class="DigNum (strict)"(reference=w383, error in=w403, "DisabledEnum"=w397) -> (error out=w402:errorcluster)  [unwired: 1 out]
            n175 = control-ref of="Range max perc."() -> (w385:refnum<vi>)
            n176 = Select(t=w386, s=w395, f=w385) -> (s? t:f=→"Range max ref":refnum<vi>)
            n177 = property class="DigNum (strict)"(reference=w385, error in=w402, "DisabledEnum"=w396) -> (error out=w401:errorcluster)  [unwired: 1 out]
            n178 = control-ref of="Range min perc."() -> (w384:refnum<vi>)
            n179 = Select(t=w383, s=w395, f=w384) -> (s? t:f=→"Range min ref":refnum<vi>)
            n180 = property class="DigNum (strict)"(reference=w384, error in=w401, "DisabledEnum"=w396) -> (error out=w393:errorcluster)  [unwired: 1 out]
            n181 = Merge Errors(w392, w393) -> (w391:errorcluster)
          }
          frame "GrabCh1Data" {
            n182 = property on="Ch1WaveformData" class="Clust (strict)"(error in=w422) -> (error out=w421:errorcluster, "Value"=w420:T2)  [unwired: 1 in, 1 out]
            n183 = property on="Datapoints ch1" class="DigNum (strict)"(error in=w421) -> (error out=w414:errorcluster, "Value"=w411:i32)  [unwired: 1 in, 1 out]
            n184 = property on="Datapoints to collect" class="DigNum (strict)"(error in=w414) -> (error out=w410:errorcluster, "Value"=w412:i32)  [unwired: 1 in, 1 out]
            n185 = Equal?(x=w412, y=w411) -> (x = y?=w413:bool)
            n186 = case shown="True" w413 {
              tunnel: w411 -> [w433 w449]
              tunnel: w420 -> [w432 _]
              tunnel: [w431 w448] -> w419
              tunnel: [w430 w449] -> w415
              tunnel: w410 -> [w429 w448]
              frame False {
                n187 = case shown="Default" w433 {
                  selector: w433 -> [w434 w446]
                  tunnel: w432 -> [w444 _]
                  tunnel: w429 -> [w437 w447]
                  tunnel: [w436 w447] -> w431
                  tunnel: [w435 w445] -> w430
                  frame Default {
                    n188 = Unbundle By Name(w444) -> ("Coincidences"=w443:dbl, "Non-coincidences"=w442:dbl)
                    n189 = property on="Data ch1" class="Arr (strict)"(error in=w437) -> (error out=w438:errorcluster, "Value"=w441:i32[][])  [unwired: 1 in, 1 out]
                    n190 = Build Array(w443, w442) -> (w440:dbl[])
                    n191 = Build Array (concatenate)(w441, w440) -> (w439:dbl[][])
                    n192 = Increment(x=w434) -> (x+1=w435:i32)
                    n193 = property on="Data ch1" class="Arr (strict)"(error in=w438, "Value"=w439) -> (error out=w436:errorcluster)  [unwired: 1 in, 1 out]
                  }
                  frame -2, -1 {
                    # "We do not record the two first data entries"
                    n194 = Increment(x=w446) -> (x+1=w445:i32)
                  }
                }
              }
              frame True {
              }
            }
            n195 = property on="Datapoints ch1" class="DigNum (strict)"(error in=w419, "Value"=w415) -> (error out=w417:errorcluster)  [unwired: 1 in, 1 out]
            n196 = property on="Datapoints ch2" class="DigNum (strict)"(error in=w417) -> (error out=w407:errorcluster, "Value"=w416:i32)  [unwired: 1 in, 1 out]
            n197 = Equal?(x=w416, y=w412) -> (x = y?=w408:bool)
            n198 = Equal?(x=w415, y=w412) -> (x = y?=w409:bool)
            n199 = And(x=w408, y=w409) -> (x .and. y?=w405:bool)
            n200 = case shown="True" w405 {
              tunnel: w407 -> [w423 w426]
              tunnel: [w423 w425] -> w406
              frame False {
              }
              frame True {
                n201 = call "Append to command queue.vi"("Name (CommandQueue)"="CoincChara", "Clear Queue (F)"=TRUE, "error in (no error)"=w426, "Single command"="LevelDone") -> ("error out"=w425:errorcluster)  [unwired: 7 in]
              }
            }
          }
          frame "GrabCh2Data" {
            n202 = property on="Ch2WaveformData" class="Clust (strict)"(error in=w467) -> (error out=w466:errorcluster, "Value"=w465:T2)  [unwired: 1 in, 1 out]
            n203 = property on="Datapoints ch2" class="DigNum (strict)"(error in=w466) -> (error out=w459:errorcluster, "Value"=w456:i32)  [unwired: 1 in, 1 out]
            n204 = property on="Datapoints to collect" class="DigNum (strict)"(error in=w459) -> (error out=w455:errorcluster, "Value"=w457:i32)  [unwired: 1 in, 1 out]
            n205 = Equal?(x=w457, y=w456) -> (x = y?=w458:bool)
            n206 = case shown="False" w458 {
              tunnel: w456 -> [w478 w494]
              tunnel: w465 -> [w477 _]
              tunnel: [w476 w493] -> w464
              tunnel: [w475 w494] -> w460
              tunnel: w455 -> [w474 w493]
              frame False {
                n207 = case shown="Default" w478 {
                  selector: w478 -> [w479 w491]
                  tunnel: w477 -> [w489 _]
                  tunnel: w474 -> [w482 w492]
                  tunnel: [w481 w492] -> w476
                  tunnel: [w480 w490] -> w475
                  frame Default {
                    n208 = Unbundle By Name(w489) -> ("Coincidences"=w488:dbl, "Non-coincidences"=w487:dbl)
                    n209 = property on="Data ch2" class="Arr (strict)"(error in=w482) -> (error out=w483:errorcluster, "Value"=w486:i32[][])  [unwired: 1 in, 1 out]
                    n210 = Build Array(w488, w487) -> (w485:dbl[])
                    n211 = Build Array (concatenate)(w486, w485) -> (w484:dbl[][])
                    n212 = Increment(x=w479) -> (x+1=w480:i32)
                    n213 = property on="Data ch2" class="Arr (strict)"(error in=w483, "Value"=w484) -> (error out=w481:errorcluster)  [unwired: 1 in, 1 out]
                  }
                  frame -2, -1 {
                    # "We do not record the two first data entries"
                    n214 = Increment(x=w491) -> (x+1=w490:i32)
                  }
                }
              }
              frame True {
              }
            }
            n215 = property on="Datapoints ch2" class="DigNum (strict)"(error in=w464, "Value"=w460) -> (error out=w462:errorcluster)  [unwired: 1 in, 1 out]
            n216 = property on="Datapoints ch1" class="DigNum (strict)"(error in=w462) -> (error out=w451:errorcluster, "Value"=w461:i32)  [unwired: 1 in, 1 out]
            n217 = Equal?(x=w461, y=w457) -> (x = y?=w453:bool)
            n218 = Equal?(x=w460, y=w457) -> (x = y?=w454:bool)
            n219 = And(x=w453, y=w454) -> (x .and. y?=w452:bool)
            n220 = case shown="True" w452 {
              tunnel: w451 -> [w468 w471]
              tunnel: [w468 w470] -> w450
              frame False {
              }
              frame True {
                n221 = call "Append to command queue.vi"("Name (CommandQueue)"="CoincChara", "Clear Queue (F)"=TRUE, "error in (no error)"=w471, "Single command"="LevelDone") -> ("error out"=w470:errorcluster)  [unwired: 7 in]
              }
            }
          }
        }
      }
      frame Error {
        w501 = "CoincChara" ("name (unnamed)")
        n222 = Obtain Queue(name (unnamed)=w501, element data type=w501) -> (queue out=w504:refnum<queue>, error out=w503:errorcluster)  [unwired: 3 in, 1 out]
        n223 = call "Append to command queue.vi"("Single command"="Stop") -> ("error out"=w496:errorcluster)  [unwired: 10 in]
        n224 = Release Queue(queue=w504, force destroy? (F)=TRUE, error in (no error)=w503) -> (error out=w500:errorcluster)  [unwired: 2 out]
        n225 = Merge Errors(w496, w500, w499) -> (w498:errorcluster)
      }
    }
    n226 = case shown="False" "generate error" {
      tunnel: [w25 errorcluster {"status"=TRUE, "code"=0, "source"=""} ("error IO")] -> w12
      tunnel: w11 -> [w25 _]
      frame False {
      }
      frame True {
      }
    }
  }
  "Error out" <- w2
